vi "findZerosInRD.vi"(9 "Probe Type":T1=12 items=["5-Hole Probe"=5, "OmniProbe"=12], 11 "Raw data file":path) -> (2 "zerosChannels":string[](array[string]))   [LabVIEW 2021]
uses:
  Controls/AeroprobeType.ctl
  f04e7692-5796-4b98-bd16-0db515aa7d3f.vi
  <vilib>/Comparison/Less/Less Functor/Less Functor.lvclass
panel:
  # "Returns the names, in correct order, of the zeros channels found in the file for the selected probe type"
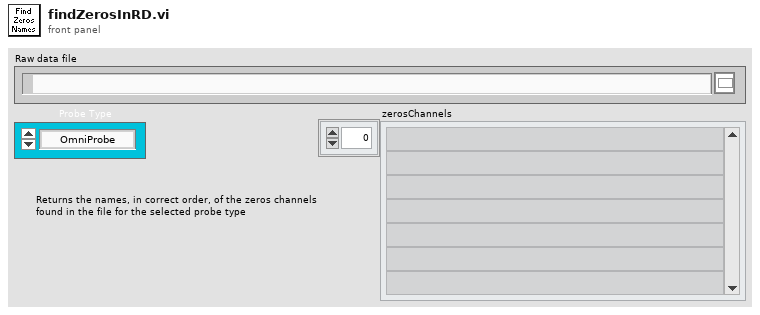
[diagram p1: front panel]
types:
  T1 = typedef "AeroprobeType.ctl" = u16
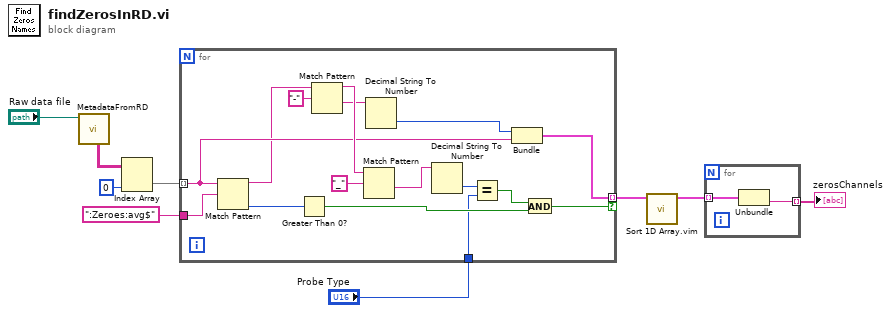
[diagram p0: block diagram]
diagram:
  n1 = call "MetadataFromRD.vi"("Raw data file"="Raw data file") -> ("Name-Value Array"=w8:string[][])  [unwired: 7 in, 3 out]
  n2 = Index Array(array=w8, index (col)=0 ("disabled index (col)")) -> (element=w6:string[])  [unwired: 1 in]
  n3 = for {
    tunnel: w6 -> [w20] mode=indexing
    tunnel: [w19] -> w5 mode=indexing if=w13
    tunnel: ":Zeroes:avg$" ("regular expression") -> [w15]
    tunnel: "Probe Type" -> [w10]
    n4 = Match Pattern(string=w20, regular expression=w15) -> (before substring=w18:string, offset past match=w25:i32)  [unwired: 1 in, 2 out]
    n5 = Greater Than 0?(x=w25) -> (x > 0?=w24:bool)
    n6 = Match Pattern(string=w18, regular expression="-") -> (before substring=w21:string, after substring=w17:string)  [unwired: 1 in, 2 out]
    n7 = Match Pattern(string=w21, regular expression="_") -> (after substring=w14:string)  [unwired: 1 in, 3 out]
    n8 = Decimal String To Number(string=w17) -> (number=w16:i32)  [unwired: 2 in, 1 out]
    n9 = Decimal String To Number(string=w14) -> (number=w11:i32)  [unwired: 2 in, 1 out]
    n10 = Equal?(x=w11, y=w10) -> (x = y?=w12:bool)
    n11 = Bundle(w16, "String"=w20) -> (w19:cluster{i32, "String":string})  [unwired: 1 in]
    n12 = And(x=w12, y=w24) -> (x .and. y?=w13:bool)
  }
  n13 = call "Sort 1D Array.vim"("unsorted array"=w5) -> ("sorted array"=w2:cluster{i32, "String":string}[])  [unwired: 10 in]
  n14 = for {
    tunnel: w2 -> [w27] mode=indexing
    tunnel: [w26] -> w1 mode=indexing
    n15 = Unbundle(w27) -> ("String"=w26:string)  [unwired: 1 out]
  }
  "zerosChannels" <- w1
